vi "Inject Attribute List.vi"(6 "Attributes Ref":refnum<data-value>, 8 "error in (no error)":errorcluster, 11 "Stop Low Pressure Wax in":refnum<class "Stop Low Pressure Wax.lvclass">) -> (0 "error out":errorcluster, 3 "Stop Low Pressure Wax out":refnum<class "Stop Low Pressure Wax.lvclass">)   [LabVIEW 2019, in "Stop Low Pressure Wax.lvclass"]
uses:
  <vilib>/gpm_packages/@cs/Car-wash/Source/Process Steps/Stop Low Pressure Wax/Stop Low Pressure Wax.lvclass
  <vilib>/gpm_packages/@cs/lookup-table/Source/LookupTable/LookupTable.lvclass
  <vilib>/gpm_packages/@cs/lookup-table/Source/LookupTable/LookupTable.lvclass/LookupTable.ctl
  <vilib>/gpm_packages/@cs/Car-wash/Source/Process Steps/Stop Low Pressure Wax/Stop Low Pressure Wax.lvclass/Stop Low Pressure Wax.ctl
  e60448ec-8064-42af-aa39-07abef02a772.vi
  <vilib>/gpm_packages/@cs/lookup-table/Source/LookupTable/Read Table Reference.vi
  e60448ec-8064-42af-aa39-07abef02a772.vi/144f6e8b-0315-407a-80b7-87f812f4395a.vi
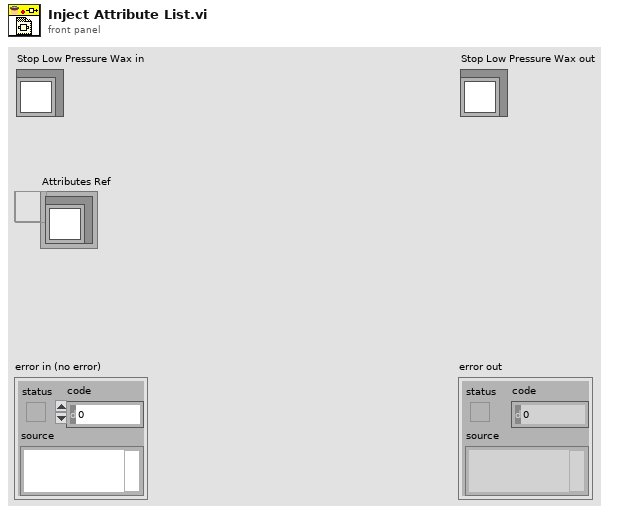
[diagram p1: front panel]
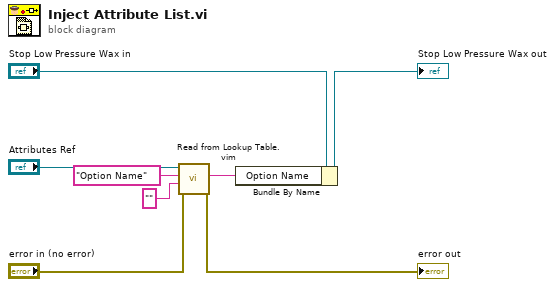
[diagram p0: block diagram]
diagram:
  n1 = call "Read from Lookup Table.vim"("error in (no error)"="error in (no error)", "Type"="", "Item Name"="Option Name", "LookupTable Reference"="Attributes Ref") -> ("error out"=→"error out":errorcluster, "Value"=w6:string)  [unwired: 4 in, 2 out]
  n2 = Bundle By Name(cluster="Stop Low Pressure Wax in", "Option Name"=w6) -> (→"Stop Low Pressure Wax out":refnum<class "Stop Low Pressure Wax.lvclass">)
